vi "XNET UDP Socket Multicast Open (Read Write).vi"(6 "local interface":string, 7 "stack":refnum<k21>, 8 "error in":errorcluster, 9 "time-to-live":u16=1, 10 "multicast address":string, 11 "local port":u16) -> (0 "error out":errorcluster, 2 "actual local port":u16, 3 "socket":refnum<k20>)   [LabVIEW 2018]
doc: "Subscribes to a UDP multicast group with read and write access on the port you specify."
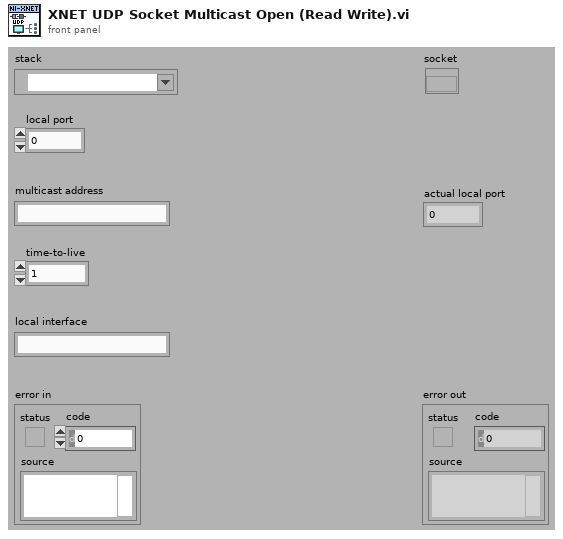
[diagram p1: front panel]
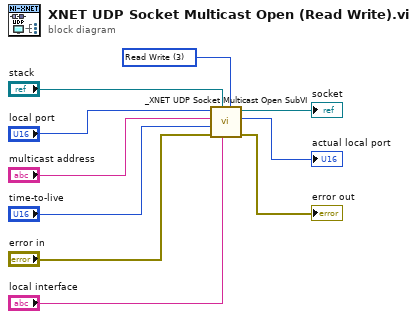
[diagram p0: block diagram]
diagram:
  w1 = u32 3 items=["Write Only"=1, "Read Only"=2, "Read Write"=3] ("mode")
  n1 = call "_XNET UDP Socket Multicast Open SubVI.vi"("mode"=w1, "local interface"="local interface", "stack"="stack", "error in"="error in", "time-to-live"="time-to-live", "multicast address"="multicast address", "local port"="local port") -> ("error out"=→"error out":errorcluster, "actual local port"=→"actual local port":u16, "socket"=→"socket":refnum<k20>)  [unwired: 2 in]
